vi "test Diff Configuration (Modify Add Remove).vi"(8 "error in":errorcluster, 11 "TestCase in":refnum<class "Refresh.lvclass">) -> (0 "error out":errorcluster, 3 "TestCase out":refnum<class "Refresh.lvclass">)   [LabVIEW 2020, in "Refresh.lvclass"]
uses:
  Refresh.lvclass
  Shared/BIU Configuration.ctl
  Shared/Address.ctl
  Shared/Major Frame Definition.ctl
  Shared/Minor Frame Definition.ctl
  Shared/Acyclic Frame Definition.ctl
  Shared/Message Definition.ctl
  Shared/Message Type.ctl
  Shared/Terminal Endpoint.ctl
  Shared/Parameter Definition.ctl
  System Explorer/Implementation/System Explorer/Refresh/MCL Row.ctl
  System Explorer/Implementation/System Explorer/Refresh/Change Type.ctl
  System Explorer/Implementation/System Explorer/Refresh/Symbols.ctl
  <vilib>/addons/_JKI Toolkits/VI Tester/TestCase.llb/TestCase.lvclass
  System Explorer/Implementation/System Explorer/Refresh/Refresh.lvlib
  C:/Program Files (x86)/National Instruments/LabVIEW 2020/vi.lib/addons/_JKI Toolkits/VI Tester/TestCase.llb/TestCase.lvclass
panel:
  out "Multicolumn Listbox":i32(listbox)=-1
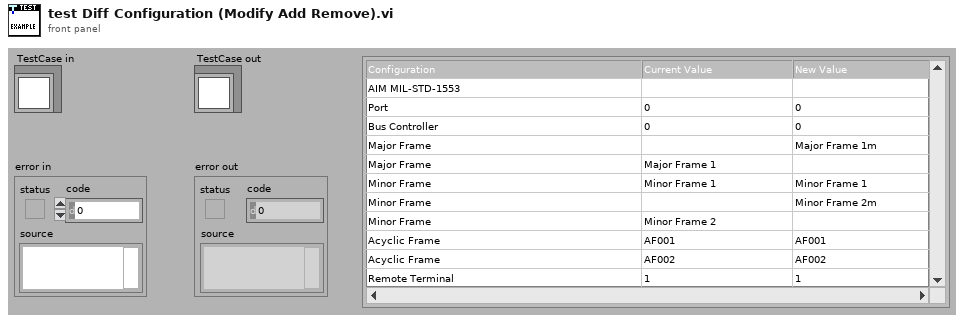
[diagram p1: front panel]
types:
  T1 = typedef "AIM MIL-STD-1553 System Explorer.lvlib/Implementation.lvlib/Refresh.lvlib/MCL Row.ctl" = cluster{"change type":T2, "item symbol":T3, "item names":string[]}
  T2 = typedef "AIM MIL-STD-1553 System Explorer.lvlib/Implementation.lvlib/Refresh.lvlib/Change Type.ctl" = enum16{"No change", "Modify", "Add", "Remove"}
  T3 = typedef "AIM MIL-STD-1553 System Explorer.lvlib/Implementation.lvlib/Refresh.lvlib/Symbols.ctl" = enum16{"Blank", "MIL-STD-1553", "Port", "Remote Terminal", "Subaddress", "Bus Controller", "Frame", "Mode Code", "Message", "Parameter", "Item"}
  T4 = typedef "BIU Configuration.ctl" = cluster{"HW channel":u16, "terminal addresses":T5[], "terminal names":string[], "major frames":T6[], "minor frames":T7[], "acyclic frames":T8[], "messages":T9[], "minor frame period (us)":i32, "starting buffer index":u16}
  T5 = typedef "Address.ctl" = u16
  T6 = typedef "Major Frame Definition.ctl" = cluster{"name":string, "minor frames":string[]}
  T7 = typedef "Minor Frame Definition.ctl" = cluster{"name":string, "messages":string[]}
  T8 = typedef "Acyclic Frame Definition.ctl" = cluster{"name":string, "messages":string[]}
  T9 = typedef "Message Definition.ctl" = cluster{"name":string, "message type":T10, "endpoint Tx":T11, "endpoint Rx":T11, "create timestamp channel":bool, "mode code":u16, "number of words":u16, "parameters":cluster{"name":string, "default value":dbl, "unit":string, "parameter definition":T12}[]}
  T10 = typedef "Message Type.ctl" = string
  T11 = typedef "Terminal Endpoint.ctl" = cluster{"terminal address":T5, "subaddress":T5}
  T12 = typedef "Parameter Definition.ctl" = cluster{"start index":i32, "size (bits)":i32, "encoding":enum16{"BNR", "BCD", "Discrete"}, "signed":bool, "multiplier":dbl, "offset":dbl}
  T13 = typedef "imagedata.ctl" = cluster{"image type":i32, "image depth":i32, "image":u8[], "mask":u8[], "colors":u32[], "Rectangle":cluster{"left":i16, "top":i16, "right":i16, "bottom":i16}}
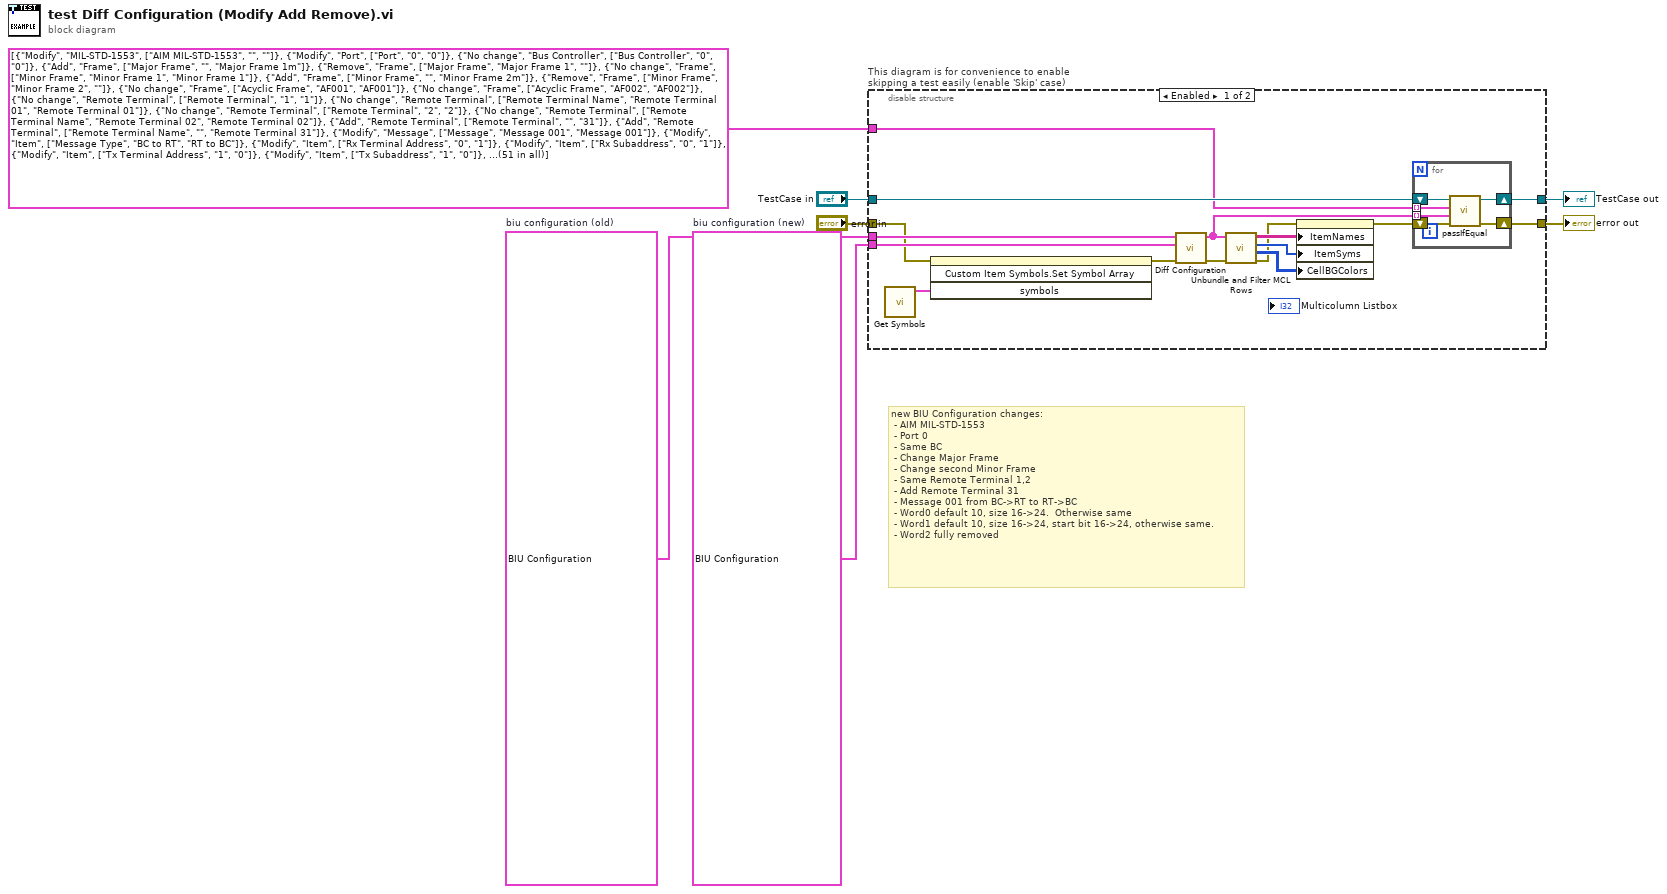
[diagram p0: block diagram]
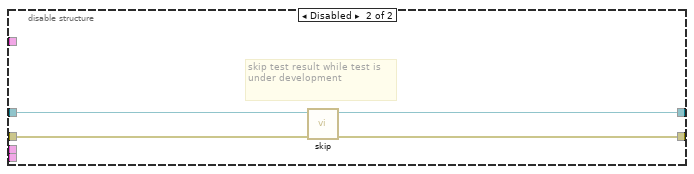
[diagram p2: hidden frame]
diagram:
  w2 = T4 {"HW channel"=0, "terminal addresses"=[0, 1, 2], "terminal names"=[], "major frames"=[{"name"="Major Frame 1", "minor frames"=[]}], "minor frames"=[{"name"="Minor Frame 1", "messages"=[]}, {"name"="Minor Frame 2", "messages"=[]}], "acyclic frames"=[{"name"="AF001", "messages"=[]}, {"name"="AF002", "messages"=[]}], "messages"=[{"name"="Message 001", "message type"="BC to RT", "endpoint Tx"={"terminal address"=1, "subaddress"=1}, "endpoint Rx"={"terminal address"=0, "subaddress"=0}, "create timestamp channel"=TRUE, "mode code"=0, "number of words"=3, "parameters"=[{"name"="Word0", "default value"=1.0, "unit"="eu", "parameter definition"={"start index"=0, "size (bits)"=16, "encoding"=enum."BNR", "signed"=FALSE, "multiplier"=1.0, "offset"=0.0}}, {"name"="Word1", "default value"=1.0, "unit"="eu", "parameter definition"={"start index"=16, "size (bits)"=16, "encoding"=enum."BNR", "signed"=TRUE, "multiplier"=1.0, "offset"=0.0}}, {"name"="Word2", "default value"=1.0, "unit"="eu", "parameter definition"={"start index"=32, "size (bits)"=16, "encoding"=enum."BNR", "signed"=TRUE, "multiplier"=1.0, "offset"=0.0}}]}], "minor frame period (us)"=0, "starting buffer index"=0}  # biu configuration (old)
  w3 = T4 {"HW channel"=0, "terminal addresses"=[0, 1, 2, 31], "terminal names"=[], "major frames"=[{"name"="Major Frame 1m", "minor frames"=[]}], "minor frames"=[{"name"="Minor Frame 1", "messages"=[]}, {"name"="Minor Frame 2m", "messages"=[]}], "acyclic frames"=[{"name"="AF001", "messages"=[]}, {"name"="AF002", "messages"=[]}], "messages"=[{"name"="Message 001", "message type"="RT to BC", "endpoint Tx"={"terminal address"=0, "subaddress"=0}, "endpoint Rx"={"terminal address"=1, "subaddress"=1}, "create timestamp channel"=TRUE, "mode code"=0, "number of words"=3, "parameters"=[{"name"="Word0", "default value"=10.0, "unit"="eu", "parameter definition"={"start index"=0, "size (bits)"=24, "encoding"=enum."BNR", "signed"=FALSE, "multiplier"=1.0, "offset"=0.0}}, {"name"="Word1", "default value"=10.0, "unit"="eu", "parameter definition"={"start index"=24, "size (bits)"=24, "encoding"=enum."BNR", "signed"=TRUE, "multiplier"=1.0, "offset"=0.0}}]}], "minor frame period (us)"=0, "starting buffer index"=0}  # biu configuration (new)
  # "new BIU Configuration changes:\n - AIM MIL-STD-1553\n - Port 0\n - Same BC\n - Change Major Frame\n - Change second Minor Frame\n - Same Remote Terminal 1,2\n - Add Remote Terminal 31\n - Message 001 from BC->RT to RT->BC\n - Word0 default 10, size 16->24.  Otherwise same\n - Word1 default 10, size 16->24, start bit 16->24, otherwise same.   \n - Word2 fully removed"
  n1 = disable-structure "This diagram is for convenience to enable skipping a test easily (enable 'Skip' case)" shown="Enabled" {
    disable-tunnel: "TestCase in" -> [w23 w33]
    disable-tunnel: [w22 w31] -> w4
    disable-tunnel: [w9 w32] -> w6
    disable-tunnel: "error in" -> [w13 w30]
    disable-tunnel: w2 -> [w21 _]
    disable-tunnel: w3 -> [w20 _]
    disable-tunnel: T1[] [{"change type"=enum."Modify", "item symbol"=enum."MIL-STD-1553", "item names"=["AIM MIL-STD-1553", "", ""]}, {"change type"=enum."Modify", "item symbol"=enum."Port", "item names"=["Port", "0", "0"]}, {"change type"=enum."No change", "item symbol"=enum."Bus Controller", "item names"=["Bus Controller", "0", "0"]}, {"change type"=enum."Add", "item symbol"=enum."Frame", "item names"=["Major Frame", "", "Major Frame 1m"]}, {"change type"=enum."Remove", "item symbol"=enum."Frame", "item names"=["Major Frame", "Major Frame 1", ""]}, {"change type"=enum."No change", "item symbol"=enum."Frame", "item names"=["Minor Frame", "Minor Frame 1", "Minor Frame 1"]}, {"change type"=enum."Add", "item symbol"=enum."Frame", "item names"=["Minor Frame", "", "Minor Frame 2m"]}, {"change type"=enum."Remove", "item symbol"=enum."Frame", "item names"=["Minor Frame", "Minor Frame 2", ""]}, {"change type"=enum."No change", "item symbol"=enum."Frame", "item names"=["Acyclic Frame", "AF001", "AF001"]}, {"change type"=enum."No change", "item symbol"=enum."Frame", "item names"=["Acyclic Frame", "AF002", "AF002"]}, {"change type"=enum."No change", "item symbol"=enum."Remote Terminal", "item names"=["Remote Terminal", "1", "1"]}, {"change type"=enum."No change", "item symbol"=enum."Remote Terminal", "item names"=["Remote Terminal Name", "Remote Terminal 01", "Remote Terminal 01"]}, {"change type"=enum."No change", "item symbol"=enum."Remote Terminal", "item names"=["Remote Terminal", "2", "2"]}, {"change type"=enum."No change", "item symbol"=enum."Remote Terminal", "item names"=["Remote Terminal Name", "Remote Terminal 02", "Remote Terminal 02"]}, {"change type"=enum."Add", "item symbol"=enum."Remote Terminal", "item names"=["Remote Terminal", "", "31"]}, {"change type"=enum."Add", "item symbol"=enum."Remote Terminal", "item names"=["Remote Terminal Name", "", "Remote Terminal 31"]}, {"change type"=enum."Modify", "item symbol"=enum."Message", "item names"=["Message", "Message 001", "Message 001"]}, {"change type"=enum."Modify", "item symbol"=enum."Item", "item names"=["Message Type", "BC to RT", "RT to BC"]}, {"change type"=enum."Modify", "item symbol"=enum."Item", "item names"=["Rx Terminal Address", "0", "1"]}, {"change type"=enum."Modify", "item symbol"=enum."Item", "item names"=["Rx Subaddress", "0", "1"]}, {"change type"=enum."Modify", "item symbol"=enum."Item", "item names"=["Tx Terminal Address", "1", "0"]}, {"change type"=enum."Modify", "item symbol"=enum."Item", "item names"=["Tx Subaddress", "1", "0"]}, {"change type"=enum."No change", "item symbol"=enum."Item", "item names"=["Number of Words", "3", "3"]}, {"change type"=enum."No change", "item symbol"=enum."Item", "item names"=["Create Timestamp Channel", "TRUE", "TRUE"]}, {"change type"=enum."No change", "item symbol"=enum."Parameter", "item names"=["Parameter", "Word0", "Word0"]}, {"change type"=enum."Modify", "item symbol"=enum."Item", "item names"=["Default Value", "1.000000", "10.000000"]}, {"change type"=enum."No change", "item symbol"=enum."Item", "item names"=["Unit", "eu", "eu"]}, {"change type"=enum."No change", "item symbol"=enum."Item", "item names"=["Start Index", "0", "0"]}, {"change type"=enum."Modify", "item symbol"=enum."Item", "item names"=["Size in Bits", "16", "24"]}, {"change type"=enum."No change", "item symbol"=enum."Item", "item names"=["Encoding", "BNR", "BNR"]}, {"change type"=enum."No change", "item symbol"=enum."Item", "item names"=["Signed", "FALSE", "FALSE"]}, {"change type"=enum."No change", "item symbol"=enum."Item", "item names"=["Scale Multiplier", "1.000000", "1.000000"]}, {"change type"=enum."No change", "item symbol"=enum."Item", "item names"=["Scale Offset", "0.000000", "0.000000"]}, {"change type"=enum."No change", "item symbol"=enum."Parameter", "item names"=["Parameter", "Word1", "Word1"]}, {"change type"=enum."Modify", "item symbol"=enum."Item", "item names"=["Default Value", "1.000000", "10.000000"]}, {"change type"=enum."No change", "item symbol"=enum."Item", "item names"=["Unit", "eu", "eu"]}, {"change type"=enum."Modify", "item symbol"=enum."Item", "item names"=["Start Index", "16", "24"]}, {"change type"=enum."Modify", "item symbol"=enum."Item", "item names"=["Size in Bits", "16", "24"]}, {"change type"=enum."No change", "item symbol"=enum."Item", "item names"=["Encoding", "BNR", "BNR"]}, {"change type"=enum."No change", "item symbol"=enum."Item", "item names"=["Signed", "TRUE", "TRUE"]}, {"change type"=enum."No change", "item symbol"=enum."Item", "item names"=["Scale Multiplier", "1.000000", "1.000000"]}, {"change type"=enum."No change", "item symbol"=enum."Item", "item names"=["Scale Offset", "0.000000", "0.000000"]}, {"change type"=enum."Remove", "item symbol"=enum."Parameter", "item names"=["Parameter", "Word2", ""]}, {"change type"=enum."Remove", "item symbol"=enum."Item", "item names"=["Default Value", "1.000000", ""]}, {"change type"=enum."Remove", "item symbol"=enum."Item", "item names"=["Unit", "eu", ""]}, {"change type"=enum."Remove", "item symbol"=enum."Item", "item names"=["Start Index", "32", ""]}, {"change type"=enum."Remove", "item symbol"=enum."Item", "item names"=["Size in Bits", "16", ""]}, {"change type"=enum."Remove", "item symbol"=enum."Item", "item names"=["Encoding", "BNR", ""]}, {"change type"=enum."Remove", "item symbol"=enum."Item", "item names"=["Signed", "TRUE", ""]}, {"change type"=enum."Remove", "item symbol"=enum."Item", "item names"=["Scale Multiplier", "1.000000", ""]}, {"change type"=enum."Remove", "item symbol"=enum."Item", "item names"=["Scale Offset", "0.000000", ""]}] ("configuration diff") -> [w19 _]
    frame Enabled {
      n2 = call "Get Symbols.vi"() -> ("MIL-STD-1553 symbols"=w14:T13[])  [unwired: 11 in]
      n3 = invoke on="Multicolumn Listbox" class="MCListbox (strict)" method="Custom Item Symbols.Set Symbol Array"(error in=w13, "symbols"=w14) -> (error out=w12:errorcluster)  [unwired: 2 in, 3 out]
      n4 = call "Diff Configuration.vi"("error in"=w12, "configuration new"=w20, "configuration old"=w21) -> ("error out"=w11:errorcluster, "configuration diff"=w8:T1[])  [unwired: 7 in]
      n5 = call "Unbundle and Filter MCL Rows.vi"("error in"=w11, "refresh items"=w8) -> ("error out"=w15:errorcluster, "background colors"=w18:u32[][], "item symbols"=w17:T3[], "item names"=w16:string[][])  [unwired: 6 in]
      n6 = property on="Multicolumn Listbox" class="MCListbox (strict)"(error in=w15, "ItemNames"=w16, "ItemSyms"=w17, "CellBGColors"=w18) -> (error out=w10:errorcluster)  [unwired: 1 in, 1 out]
      n7 = for {
        tunnel: w19 -> [w27] mode=indexing
        tunnel: w8 -> [w26] mode=indexing
        shift-right: [w28] -> w22
        shift-left: w23 -> [w29]
        shift-right: [w24] -> w9
        shift-left: w10 -> [w25]
        n8 = call-dynamic "passIfEqual.vi"("error in (no error)"=w25, "y"=w26, "x"=w27, "TestCase in"=w29) -> ("error out"=w24:errorcluster, "TestCase out"=w28:refnum<class "Refresh.lvclass">)  [unwired: 6 in]
      }
    }
    frame Disabled {
      # "skip test result while test is under development"
      n9 = call <vilib>:"skip.vi"("error in (no error)"=w30, "TestCase in"=w33) -> ("error out"=w32:errorcluster, "TestCase out"=w31:refnum<class "Refresh.lvclass">)  [unwired: 8 in]
    }
  }
  "error out" <- w6
  "TestCase out" <- w4
